vi "Check Leap Driver.vi"(8 "Error In":errorcluster) -> (0 "Error Out":errorcluster, 2 "Installed?":bool)   [LabVIEW 2014, in "LMH-Leap.lvlib"]
uses:
  LMH-Leap.lvlib
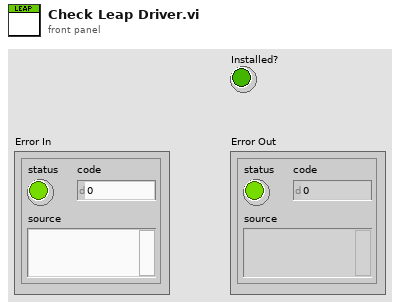
[diagram p1: front panel]
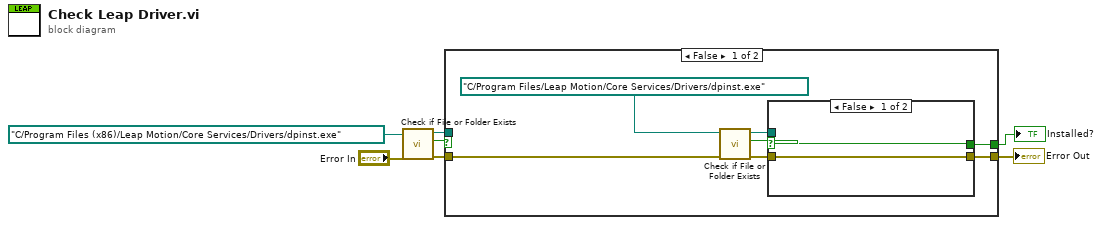
[diagram p0: block diagram]
diagram:
  n1 = call <vilib>:"Check if File or Folder Exists.vi"("error in (no error)"="Error In", "path"=path "C:/Program Files (x86)/Leap Motion/Core Services/Drivers/dpinst.exe") -> ("error out"=w4:errorcluster, "file or folder exists?"=w6:bool, "dup path"=w5:path)  [unwired: 7 in]
  n2 = case shown="False" w6 {
    selector: w6 -> [_ w19]
    tunnel: w5 -> [_ _]
    tunnel: w4 -> [w13 w20]
    tunnel: [w9 w20] -> w2
    tunnel: [w8 w19] -> w1
    frame False {
      n3 = call <vilib>:"Check if File or Folder Exists.vi"("error in (no error)"=w13, "path"=path "C:/Program Files/Leap Motion/Core Services/Drivers/dpinst.exe") -> ("error out"=w10:errorcluster, "file or folder exists?"=w11:bool, "dup path"=w12:path)  [unwired: 7 in]
      n4 = case shown="False" w11 {
        selector: w11 -> [w15 w17]
        tunnel: w12 -> [_ _]
        tunnel: w10 -> [w16 w18]
        tunnel: [w16 w18] -> w9
        tunnel: [w15 w17] -> w8
        frame False {
        }
        frame True {
        }
      }
    }
    frame True {
      # "Insalled under (x86)"
    }
  }
  "Error Out" <- w2
  "Installed?" <- w1
